vi "StagePauseTest.vi"() -> ()   [LabVIEW 2016]
panel:
  in  "completed":bool
  in  "terminate":bool
  in  "pause":bool
  in  "Axis Speeds":T1={"vX [mm/s]"=25.0, "vY [mm/s]"=12.5, "vZ [mm/s]"=5.0}
  in  "Go to Coordinates":T2={"X [mm]"=25.0, "Y [mm]"=12.5, "Z [mm]"=5.0}
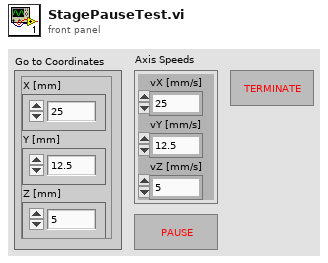
[diagram p1: front panel]
types:
  T1 = cluster{"vX [mm/s]":dbl, "vY [mm/s]":dbl, "vZ [mm/s]":dbl}
  T2 = cluster{"X [mm]":dbl, "Y [mm]":dbl, "Z [mm]":dbl}
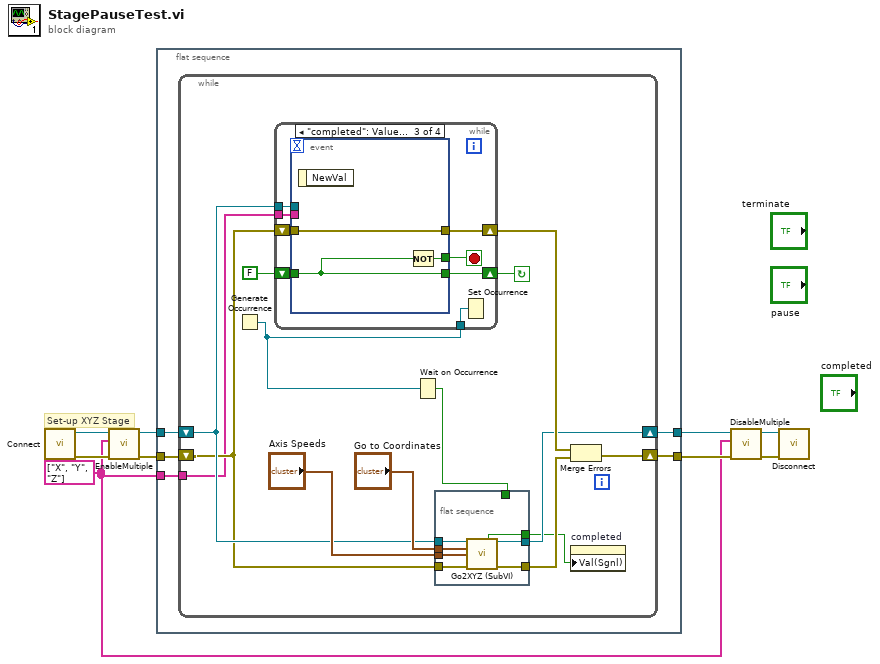
[diagram p0: block diagram]
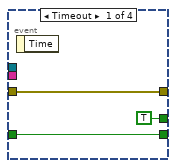
[diagram p2: hidden frame]
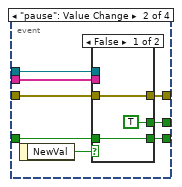
[diagram p3: hidden frame]
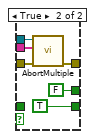
[diagram p4: hidden frame]
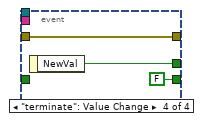
[diagram p5: hidden frame]
diagram:
  w2 = string[] ["X", "Y", "Z"] ("axis names")
  # "Set-up XYZ Stage"
  n1 = call "Connect.vi"() -> ("error out"=w9:errorcluster, "controller"=w8:refnum<k24>)  [unwired: 10 in]
  n2 = call "EnableMultiple.vi"("error in (no error)"=w9, "axis names"=w2, "controller in"=w8) -> ("error out"=w4:errorcluster, "controller out"=w1:refnum<k24>)  [unwired: 7 in]
  n3 = flat-sequence {
    tunnel: w1 -> [w14]
    tunnel: [w10] -> w5
    tunnel: w4 -> [w13]
    tunnel: [w11] -> w3
    tunnel: w2 -> [w12]
    frame #0 {
      n4 = while {
        tunnel: w12 -> [w24]
        shift-right: [w20] -> w10
        shift-left: w14 -> [w26]
        shift-right: [w23] -> w11
        shift-left: w13 -> [w25]
        stop <- w18 continue-if-true
        n5 = Generate Occurrence() -> (w16:refnum<k4>)
        n6 = while {
          shift-right: [w43] -> w21
          shift-left: w25 -> [w40]
          tunnel: w26 -> [w41]
          tunnel: w24 -> [w42]
          shift-right: [w39] -> w18
          shift-left: FALSE -> [w38]
          tunnel: w16 -> [w36]
          stop <- w37 stop-if-true
          n7 = event shown="[2] \"completed\": Value Change" {
            selector: _ -> [_ _ _ _]
            dyn-events: _ -> [_ _ _ _]
            timeout: _ -> [_ _ _ _]
            tunnel: [w46 w54 w66 w68] -> w43
            tunnel: w42 -> [_ w53 _ _]
            tunnel: w41 -> [_ w52 _ _]
            tunnel: w40 -> [w46 w51 w66 w68]
            tunnel: [w45 w49 w64 FALSE] -> w39
            tunnel: w38 -> [w45 w48 w64 _]
            tunnel: [TRUE ("NewVal") w47 w65 w69] -> w37
            event Timeout {
              n8 = event-data() -> ()  [unwired: 1 in, 1 out]
            }
            event "pause": Value Change {
              n9 = event-data() -> ("NewVal"=w50:bool)  [unwired: 1 in]
              n10 = case shown="False" w50 {
                tunnel: [w56 w63] -> w54
                tunnel: w53 -> [_ w62]
                tunnel: w52 -> [_ w61]
                tunnel: w51 -> [w56 w60]
                tunnel: [w57 TRUE] -> w49
                tunnel: w48 -> [w57 _]
                tunnel: [TRUE ("NewVal") FALSE ("NewVal")] -> w47
                frame False {
                }
                frame True {
                  n11 = call "AbortMultiple.vi"("error in (no error)"=w60, "axis names"=w62, "controller in"=w61) -> ("error out"=w63:errorcluster)  [unwired: 7 in, 1 out]
                }
              }
            }
            event "completed": Value Change {
              n12 = event-data() -> ()  [unwired: 1 in, 1 out]
              n13 = Not(x=w64) -> (.not. x?=w65:bool)
            }
            event "terminate": Value Change {
              n14 = event-data() -> ("NewVal"=w69:bool)  [unwired: 1 in]
            }
          }
          n15 = Set Occurrence(w36) -> ()
        }
        n16 = Wait on Occurrence(2:w16) -> (0:w15:bool)  [unwired: 2 in]
        n17 = flat-sequence {
          tunnel: "Axis Speeds" -> [w35]
          tunnel: "Go to Coordinates" -> [w34]
          tunnel: w26 -> [w33]
          tunnel: w25 -> [w32]
          tunnel: [w31] -> w22
          tunnel: [w30] -> w20
          tunnel: [w29] -> w17
          tunnel: w15 -> [_]
          frame #0 {
            n18 = call "Go2XYZ (SubVI).vi"(".NET Refnum in"=w33, "Go to Coordinates"=w34, "Axis Speeds"=w35, "error in (no error)"=w32) -> ("completed"=w29:bool, ".NET Refnum out"=w30:refnum<k24>, "error out"=w31:errorcluster)  [unwired: 7 in, 2 out]
          }
        }
        n19 = Merge Errors(w21, w22) -> (w23:errorcluster)
        n20 = property on="completed" class="Bool (strict)"("Val(Sgnl)"=w17) -> ()  [unwired: 2 in, 2 out]
      }
    }
  }
  n21 = call "DisableMultiple.vi"("error in (no error)"=w3, "axis names"=w2, "controller in"=w5) -> ("error out"=w6:errorcluster, "controller out"=w7:refnum<k24>)  [unwired: 7 in]
  n22 = call "Disconnect.vi"("error in (no error)"=w6, "controller"=w7) -> ()  [unwired: 9 in, 1 out]
